vi "Enumerate.vi"(6 "Postfix pattern":string="::INSTR", 7 "Prefix pattern":string="USB?*::0x1BFA::0x0498::", 8 "Error in (no error)":errorcluster, 9 "Serial No Pattern":string="%x", 10 "S/N Offset":u32=22, 11 "Serial number":string) -> (0 "Error out":errorcluster, 1 "Index":u16, 2 "Serial numbers":string[](array[string]), 3 "VISA resource":refnum<visa-resource-name>)   [LabVIEW 2010]
doc: "Copyright (c) 2012 Metrolab Technology SA, Plan-les-Ouates, Geneva, Switzerland\nEnumerate the VISA resource names of the instruments currently connected. The resource names must be some pattern (\"Prefix pattern\"), followed by the instrument's serial number, followed by another pattern (\"Postfix pattern\"). If the currently selected instrument is still connected, its index in the list is returned; else an index of zero is returned."
uses:
  <vilib>/Instr/_visa.llb/VISA Find Search Mode.ctl
panel:
  # "Enumerate"
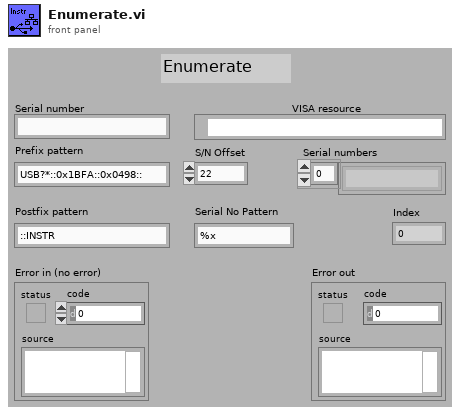
[diagram p1: front panel]
types:
  T1 = typedef "VISA Find Search Mode.ctl" = u32
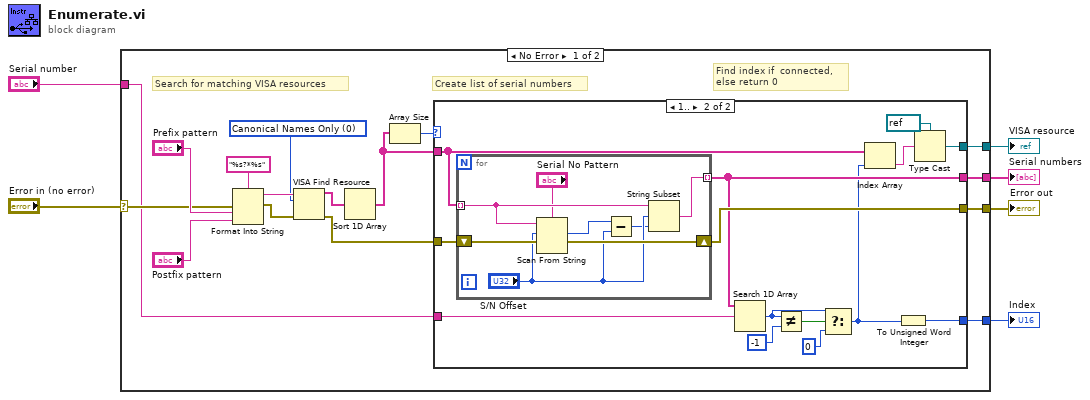
[diagram p0: block diagram]
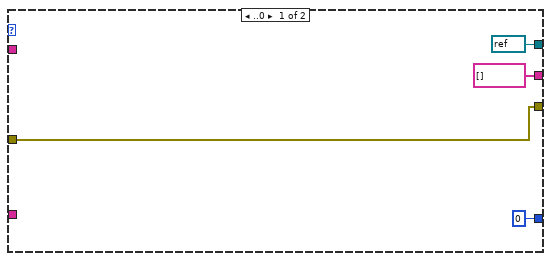
[diagram p2: hidden frame]
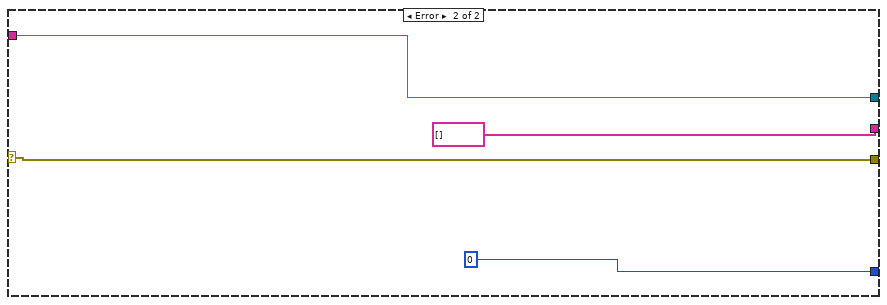
[diagram p3: hidden frame]
diagram:
  n1 = case shown="No Error" "Error in (no error)" {
    selector: "Error in (no error)" -> [w20 w52]
    tunnel: [w14 w52] -> w5
    tunnel: [w11 u16 0 ("Serial number")] -> w4
    tunnel: [w12 string[] []] -> w1
    tunnel: "Serial number" -> [w13 w49]
    tunnel: [w10 w49] -> w2
    frame No Error {
      w7 = T1 0 items=["Canonical Names Only"=0, "Aliases Only"=2, "Include Matching Aliases"=3, "Include All Aliases"=4] ("Search Mode")
      # "Find index if  connected,\nelse return 0"
      # "Search for matching VISA resources"
      # "Create list of serial numbers"
      n2 = Format Into String(format string="%s?*%s", error in=w20, "Prefix pattern", "Postfix pattern") -> (resulting string=w19:string, error out=w18:errorcluster)  [unwired: 1 in]
      n3 = VISA Find Resource(8:w18, 10:w7, 11:w19) -> (0:w15:errorcluster, 3:w16:string[])  [unwired: 1 out]
      n4 = Sort 1D Array(array=w16) -> (sorted array=w9:string[])
      n5 = Array Size(array=w9) -> (size(s)=w8:i32)
      n6 = case shown="1.." w8 {
        tunnel: w15 -> [w24 w40]
        tunnel: [w24 w39] -> w14
        tunnel: w13 -> [_ w34]
        tunnel: w9 -> [_ w33]
        tunnel: [string[] [] w32] -> w12
        tunnel: [u16 0 ("t") w27] -> w11
        tunnel: [refnum<visa-resource-name> refnum ("VISA resource") w30] -> w10
        frame ..0 {
        }
        frame 1.. {
          n7 = for {
            tunnel: w33 -> [w43] mode=indexing
            tunnel: [w42] -> w32 mode=indexing
            shift-right: [w48] -> w39
            shift-left: w40 -> [w47]
            n8 = Scan From String(format string="Serial No Pattern", input string=w43, initial scan location="S/N Offset", error in=w47) -> (offset past scan=w44:u32, error out=w48:errorcluster)  [unwired: 2 in, 1 out]
            n9 = Subtract(x=w44, y="S/N Offset") -> (x-y=w45:u32)
            n10 = String Subset(string=w43, offset (0)="S/N Offset", length (rest)=w45) -> (substring=w42:string)
          }
          n11 = Search 1D Array(1D array=w32, element=w34) -> (index of element=w35:i32)  [unwired: 1 in]
          n12 = Not Equal?(x=w35, y=-1) -> (x != y?=w37:bool)
          n13 = Select(t=w35, s=w37, f=0 ("t")) -> (s? t:f=w31:i32)
          n14 = Index Array(array=w33, index=w31) -> (element=w29:string)
          n15 = To Unsigned Word Integer(number=w31) -> (unsigned 16bit integer=w27:u16)
          n16 = Type Cast(type=refnum<visa-resource-name> refnum ("VISA resource"), x=w29) -> (*(type *) &x=w30:refnum<visa-resource-name>)
        }
      }
    }
    frame Error {
    }
  }
  "Error out" <- w5
  "Index" <- w4
  "VISA resource" <- w2
  "Serial numbers" <- w1
